vi "BUFF_POLICY - Type.vi"(8 "error in (no error)":errorcluster, 11 "BUFF_POLICY":T1=enum."SAFE") -> (0 "error out":errorcluster, 3 "BUFF_POLICY_VALUE":i32)   [LabVIEW 2015]
doc: "<b>Buffer policy settings can be only safe in xiAPI LabVIEW library</b>\nUNSAFE : User gets pointer to internally allocated circle buffer and data may be overwritten by device.\nSAFE : Data from device will be copied to user allocated buffer or xiApi allocated memory."
uses:
  C:/GIT/Cameras3.x/Integrations/Labview/xiLib/xiLIB_32bit/xiLIB/xiCamLib/API/x86/xiApi.NET.dll
  xiLIB_32bit/xiLIB/xiCamLib/API/x86/xiApi.NET.dll
  BUFF_POLICY.ctl
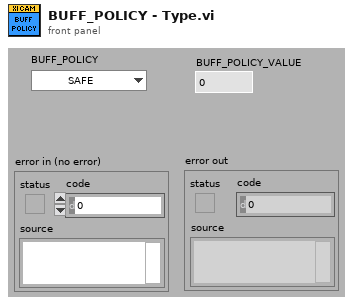
[diagram p1: front panel]
types:
  T1 = typedef "BUFF_POLICY.ctl" = enum16{"UNSAFE", "SAFE"}
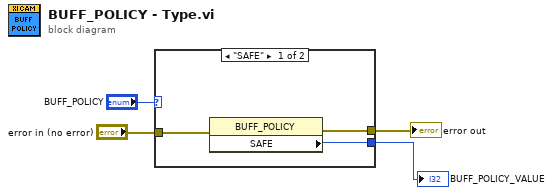
[diagram p0: block diagram]
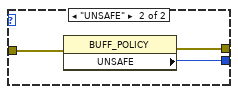
[diagram p2: hidden frame]
diagram:
  n1 = case shown="\"SAFE\"" "BUFF_POLICY" {
    tunnel: "error in (no error)" -> [w7 w10]
    tunnel: [w6 w9] -> w2
    tunnel: [w5 w8] -> w1
    frame "SAFE" {
      n2 = property class="BUFF_POLICY"(error in=w7) -> (error out=w6:errorcluster, "SAFE"=w5:i32)  [unwired: 1 in, 1 out]
    }
    frame "UNSAFE" {
      n3 = property class="BUFF_POLICY"(error in=w10) -> (error out=w9:errorcluster, "UNSAFE"=w8:i32)  [unwired: 1 in, 1 out]
    }
  }
  "error out" <- w2
  "BUFF_POLICY_VALUE" <- w1
